vi "sub4.vi"(11 "Terminal in":refnum<vi>) -> (3 "Argument":T1)   [LabVIEW 2020, in "CSM-Helper.lvclass"]
uses:
  CSM-Helper.lvclass
  Typedef/Def-Argument Info.ctl
  <userlib>/_NEVSTOP/Communicable State Machine(CSM)/Communicable State Machine.lvlib
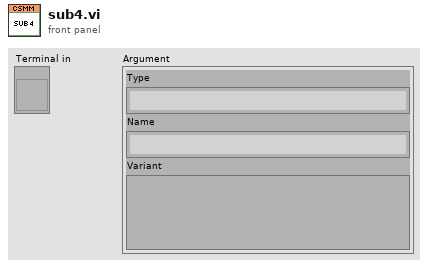
[diagram p1: front panel]
types:
  T1 = typedef "CSM-Helper.lvclass/Def-Argument Info.ctl" = cluster{"Type":string, "Name":string, "Variant":variant}
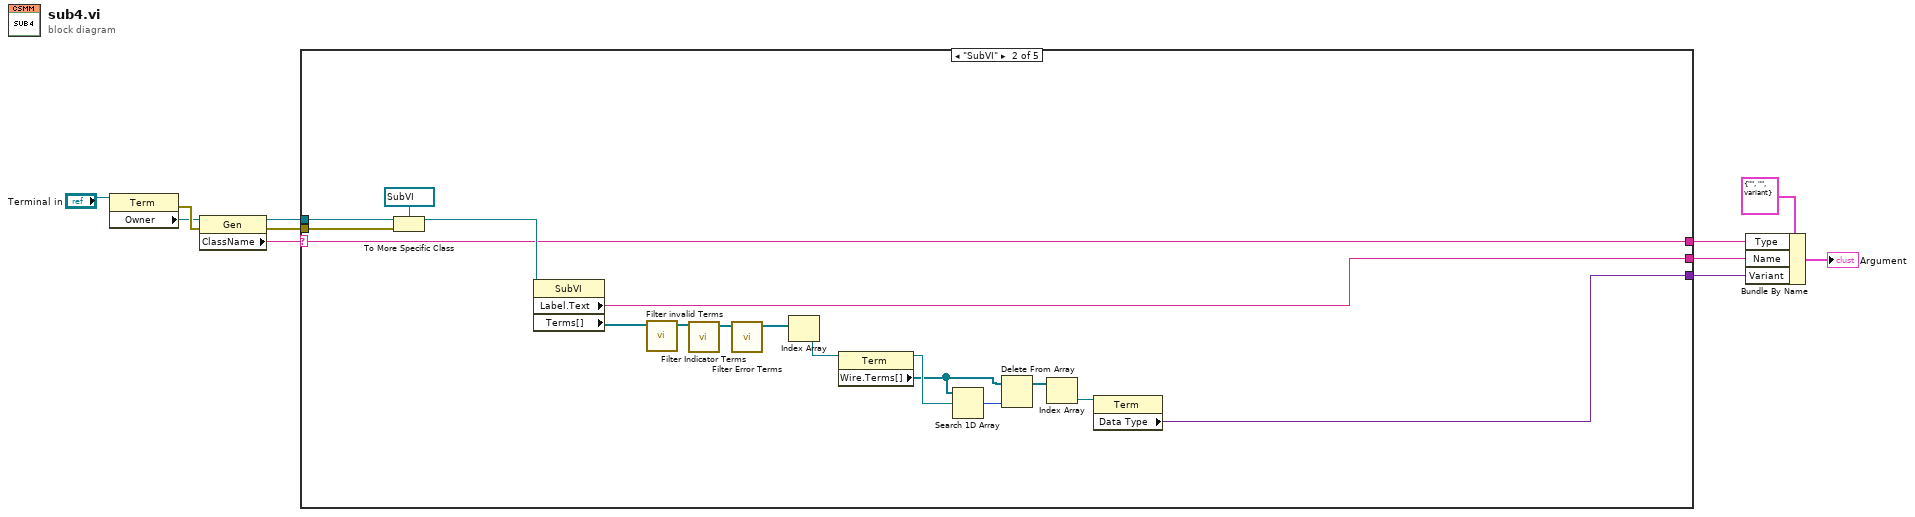
[diagram p0: block diagram]
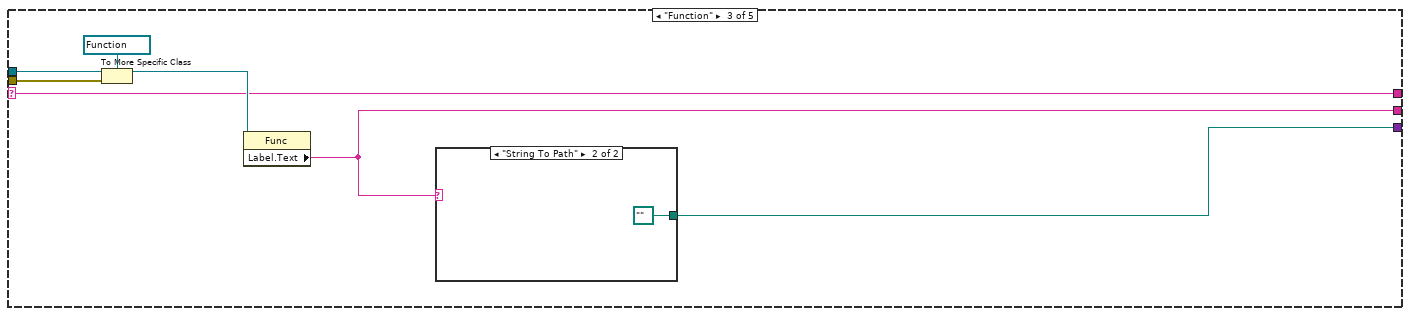
[diagram p3: hidden frame]
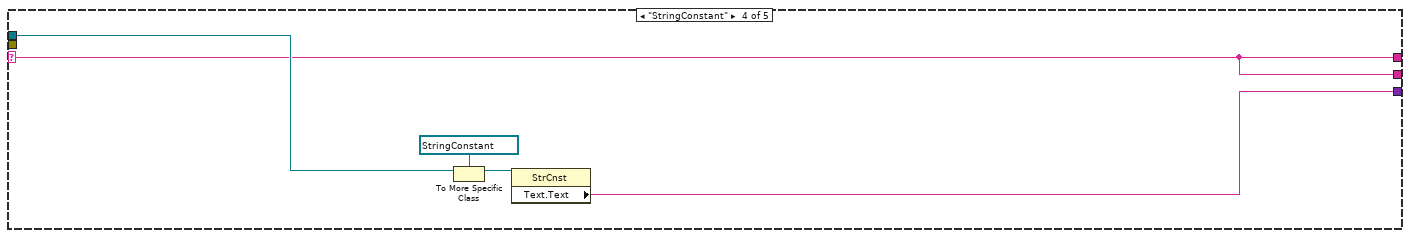
[diagram p5: hidden frame]
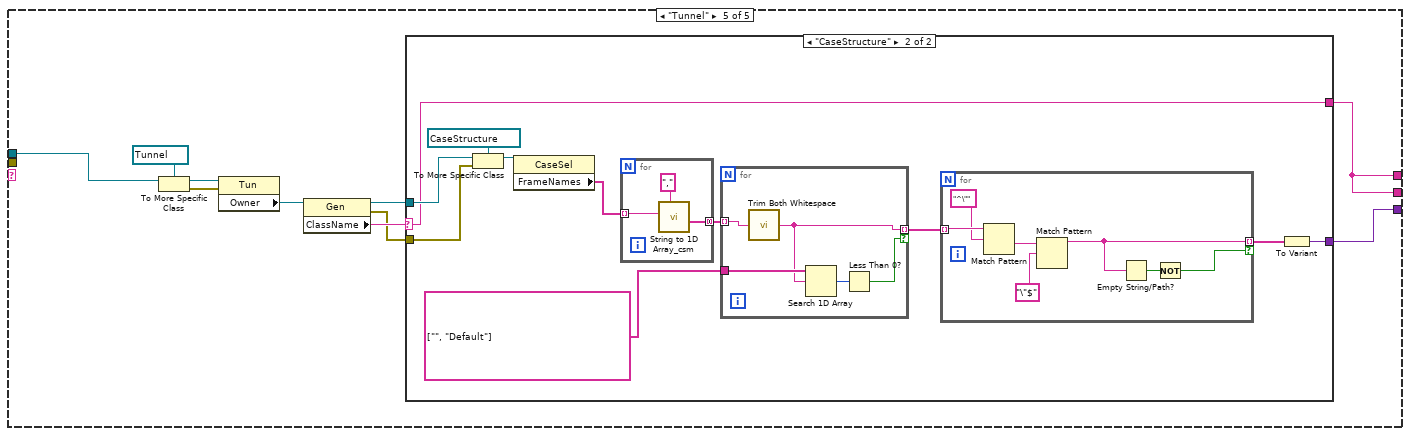
[diagram p6: hidden frame]
diagram:
  n1 = property class="Term"(reference="Terminal in") -> (error out=w6:errorcluster, "Owner"=w4:refnum<vi>)  [unwired: 1 in, 1 out]
  n2 = property class="Gen"(reference=w4, error in=w6) -> (reference out=w5:refnum<vi>, error out=w1:errorcluster, "ClassName"=w8:string)
  n3 = case shown="\"SubVI\"" w8 {
    selector: w8 -> [w12 w25 w33 w38 _]
    tunnel: w5 -> [_ w27 w34 w40 w51]
    tunnel: [_ w26 w31 w38 w43] -> w9
    tunnel: [_ w13 w30 w39 w52] -> w10
    tunnel: [w12 w25 w33 w38 w43] -> w2
    tunnel: w1 -> [_ w24 w32 _ _]
    frame Default {
    }
    frame "SubVI" {
      n4 = To More Specific Class(target class=refnum<vi> refnum ("reference out"), reference=w27, error in=w24) -> (specific class reference=w28:refnum<vi>)  [unwired: 1 out]
      n5 = property class="SubVI"(reference=w28) -> ("Label.Text"=w26:string, "Terms[]"=w21:refnum<vi>[])  [unwired: 1 in, 2 out]
      n6 = call "Filter invalid Terms.vi"("Terms[]"=w21) -> ("Terms[] out"=w22:refnum<vi>[])  [unwired: 10 in]
      n7 = call "Filter Indicator Terms.vi"("Terms[]"=w22) -> ("Terms[] out"=w23:refnum<vi>[])  [unwired: 10 in]
      n8 = call "Filter Error Terms.vi"("Terms[]"=w23) -> ("Terms[] out"=w20:refnum<vi>[])  [unwired: 10 in]
      n9 = Index Array(array=w20) -> (element=w19:refnum<vi>)  [unwired: 1 in]
      n10 = property class="Term"(reference=w19) -> (reference out=w18:refnum<vi>, "Wire.Terms[]"=w16:refnum<vi>[])  [unwired: 1 in, 1 out]
      n11 = Search 1D Array(1D array=w16, element=w18) -> (index of element=w17:i32)  [unwired: 1 in]
      n12 = Delete From Array(array=w16, index=w17) -> (array with subset deleted=w15:refnum<vi>[])  [unwired: 1 in, 1 out]
      n13 = Index Array(array=w15) -> (element=w14:refnum<vi>)  [unwired: 1 in]
      n14 = property class="Term"(reference=w14) -> ("Data Type"=w13:variant)  [unwired: 1 in, 2 out]
    }
    frame "Function" {
      n15 = To More Specific Class(target class=refnum<vi> refnum ("reference out"), reference=w34, error in=w32) -> (specific class reference=w35:refnum<vi>)  [unwired: 1 out]
      n16 = property class="Func"(reference=w35) -> ("Label.Text"=w31:string)  [unwired: 1 in, 2 out]
      n17 = case shown="\"String To Path\"" w31 {
        tunnel: [_ path ""] -> w30
        frame "False", Default {
        }
        frame "String To Path" {
        }
      }
    }
    frame "StringConstant" {
      n18 = To More Specific Class(target class=refnum<vi> refnum ("reference out"), reference=w40) -> (specific class reference=w42:refnum<vi>)  [unwired: 1 in, 1 out]
      n19 = property class="StrCnst"(reference=w42) -> ("Text.Text"=w39:string)  [unwired: 1 in, 2 out]
    }
    frame "Tunnel" {
      n20 = To More Specific Class(target class=refnum<vi> refnum ("reference out"), reference=w51) -> (specific class reference=w49:refnum<vi>, error out=w48:errorcluster)  [unwired: 1 in]
      n21 = property class="Tun"(reference=w49, error in=w48) -> ("Owner"=w47:refnum<vi>)  [unwired: 2 out]
      n22 = property class="Gen"(reference=w47) -> (reference out=w45:refnum<vi>, error out=w44:errorcluster, "ClassName"=w46:string)  [unwired: 1 in]
      n23 = case shown="\"CaseStructure\"" w46 {
        selector: w46 -> [w53 w57]
        tunnel: [_ w60] -> w52
        tunnel: w45 -> [_ w59]
        tunnel: w44 -> [_ w58]
        tunnel: [w53 w57] -> w43
        frame Default {
        }
        frame "CaseStructure" {
          n24 = To More Specific Class(target class=refnum<vi> refnum ("reference out"), reference=w59, error in=w58) -> (specific class reference=w64:refnum<vi>)  [unwired: 1 out]
          n25 = property class="CaseSel"(reference=w64) -> ("FrameNames"=w61:string[])  [unwired: 1 in, 2 out]
          n26 = for {
            tunnel: [w71] -> w62 mode=concatenating
            tunnel: w61 -> [w70] mode=indexing
            n27 = call <userlib>:"String to 1D Array_csm.vi"("delimiter (Tab)"=",", "string"=w70) -> ("Array of Strings"=w71:string[])  [unwired: 9 in]
          }
          n28 = for {
            tunnel: [w67] -> w54 mode=indexing if=w65
            tunnel: w62 -> [w69] mode=indexing
            tunnel: string[] ["", "Default"] ("items to filter") -> [w68]
            n29 = call <userlib>:"Trim Both Whitespace.vi"("string"=w69) -> ("trimmed string"=w67:string)  [unwired: 1 in]
            n30 = Search 1D Array(1D array=w68, element=w67) -> (index of element=w66:i32)  [unwired: 1 in]
            n31 = Less Than 0?(x=w66) -> (x < 0?=w65:bool)
          }
          n32 = for {
            tunnel: w54 -> [w79] mode=indexing
            tunnel: [w75] -> w56 mode=indexing if=w74
            n33 = Match Pattern(string=w79, regular expression="^\"") -> (after substring=w77:string)  [unwired: 1 in, 3 out]
            n34 = Match Pattern(string=w77, regular expression="\"$") -> (before substring=w75:string)  [unwired: 1 in, 3 out]
            n35 = Empty String/Path?(string/path=w75) -> (empty?=w73:bool)
            n36 = Not(x=w73) -> (.not. x?=w74:bool)
          }
          n37 = To Variant(anything=w56) -> (Variant=w60:variant)
        }
      }
    }
  }
  n38 = Bundle By Name(cluster=T1 {"Type"="", "Name"="", "Variant"=variant} ("Argument"), "Type"=w2, "Name"=w9, "Variant"=w10) -> (→"Argument":T1)
